vi "GetName.vi"(8 "error in (no error)":errorcluster, 11 "National Instruments USB-8473 Adapter Class in":refnum<class "National Instruments USB-8473 Adapter Class.lvclass">) -> (0 "error out":errorcluster, 2 "Value":string, 3 "National Instruments USB-8473 Adapter Class out":refnum<class "National Instruments USB-8473 Adapter Class.lvclass">)   [LabVIEW 2011, in "National Instruments USB-8473 Adapter Class.lvclass"]
uses:
  National Instruments USB-8473 Adapter Class.lvclass
  Generic CAN Adapter/GenericCanAdapterClass.lvclass
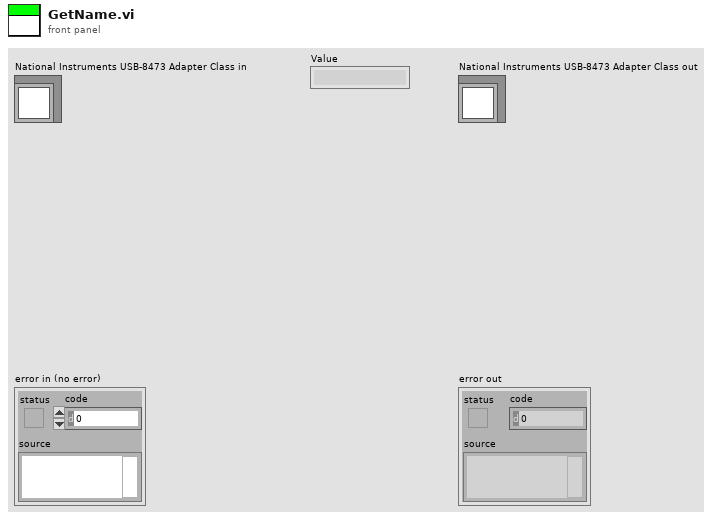
[diagram p1: front panel]
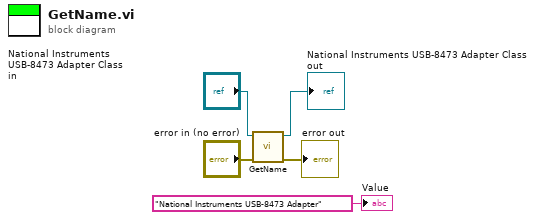
[diagram p0: block diagram]
diagram:
  n1 = call-parent "GetName.vi"("error in (no error)"="error in (no error)", "GenericCanAdapterClass in"="National Instruments USB-8473 Adapter Class in") -> ("error out"=→"error out":errorcluster, "GenericCanAdapterClass out"=→"National Instruments USB-8473 Adapter Class out":refnum<class "National Instruments USB-8473 Adapter Class.lvclass">)  [unwired: 7 in, 1 out]
  "Value" <- "National Instruments USB-8473 Adapter" ("Value")
